vi "FG_FPGA_Interface.vi"(7 "Action":T1, 8 "error in":errorcluster) -> (0 "error out":errorcluster, 3 "FPGA VI Reference Out":refnum<k20>)   [LabVIEW 2014]
uses:
  Typedef_FPGA_Interface_Action.ctl
  <vilib>/FPGAPlugInAG/cRIO-9068/niLvFpga_Open_cRIO-9068.vi
  <vilib>/rvi/interface/common/dynamic/niFpgaDynamicAddResources.vi
  <vilib>/Utility/error.llb/Error Cluster From Error Code.vi
  <vilib>/rvi/errors/niLvFpgaAdjustHostInterfaceError.vi
  <vilib>/nisyscfg/Initialize (Control).vi
  <vilib>/nisyscfg/Find Hardware.vi
  <vilib>/FPGAPlugInAG/Dynamic/niLvFpga_Close_Dynamic.vi
  <vilib>/rvi/interface/nirviOpenFPGA/nirviOpenFPGA.xnode
  FPGA Bitfiles/Main FPGA 5-axis for Candy Packaging.lvbitx
  <vilib>/rvi/interface/nirviReadWriteControl/nirviReadWriteControl.xnode
  <vilib>/rvi/interface/nirviCloseFPGA/nirviCloseFPGA.xnode
  <vilib>/nisyscfg/nisyscfg.lvlib
  <vilib>/rvi/interface/Simulation/niFpgaSimulationCallBeginRW.vi
  NiFpgaLv.dll
panel:
  out "Numeric":i32
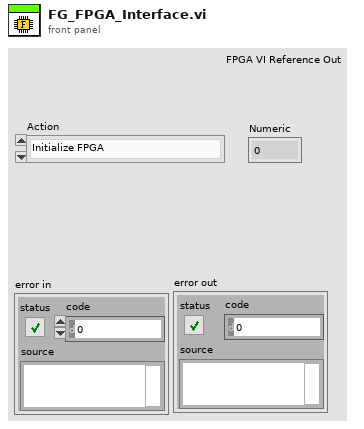
[diagram p1: front panel]
types:
  T1 = typedef "Typedef_FPGA_Interface_Action.ctl" = enum16{"Initialize FPGA", "Get FPGA Reference", "Close FPGA"}
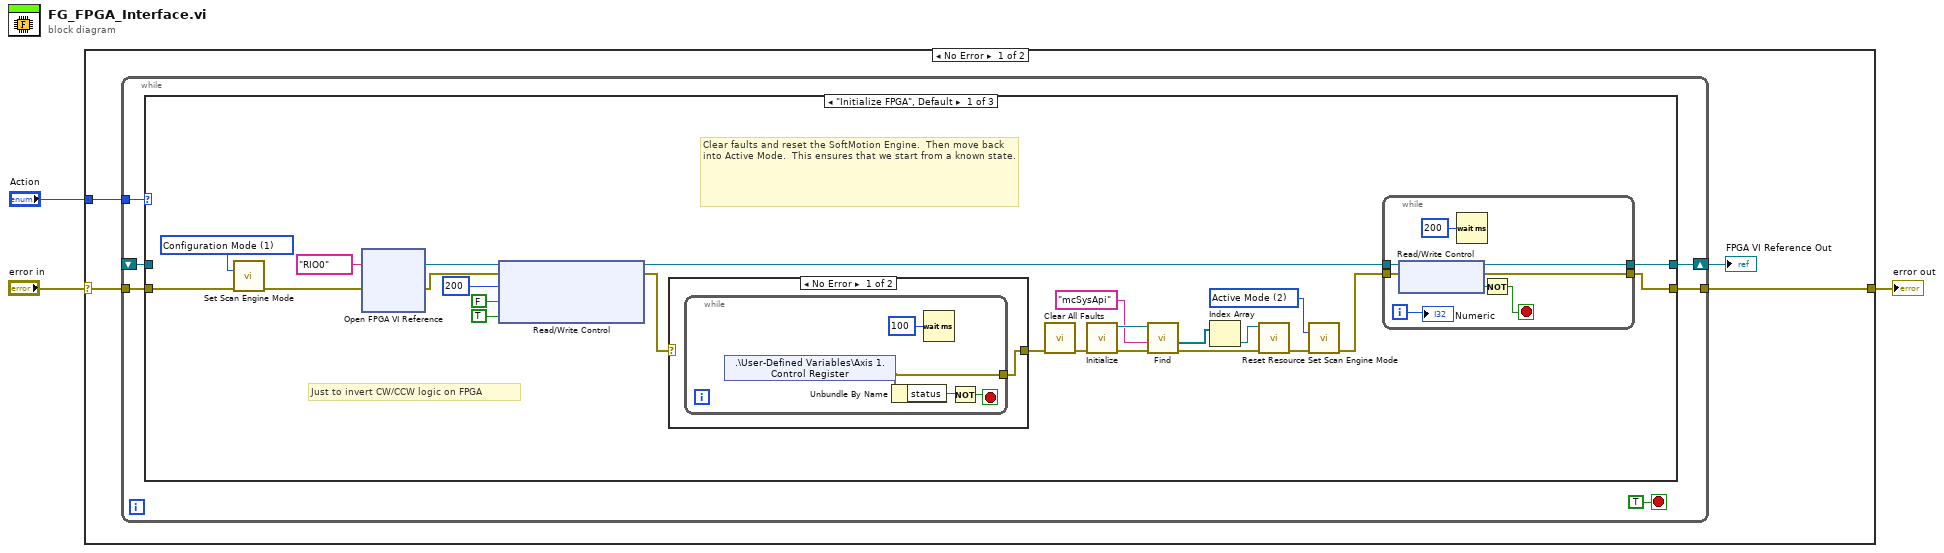
[diagram p0: block diagram]
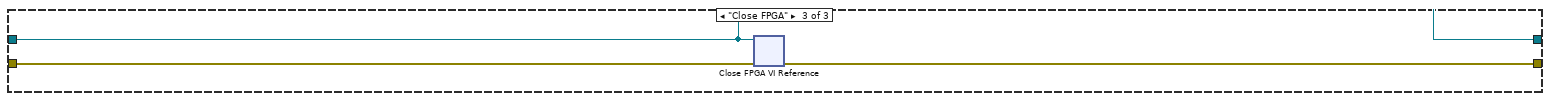
[diagram p4: hidden frame]
diagram:
  n1 = case shown="No Error" "error in" {
    selector: "error in" -> [w7 w57]
    tunnel: [w6 w57] -> w2
    tunnel: "Action" -> [w5 _]
    frame No Error {
      n2 = while {
        tunnel: w7 -> [w11]
        tunnel: w5 -> [w12]
        tunnel: [w10] -> w6
        shift-right: [w9] -> w4
        shift-left: _ -> [w8]
        stop <- TRUE stop-if-true
        n3 = case shown="\"Initialize FPGA\", Default" w12 {
          tunnel: w11 -> [w36 w52 w55]
          tunnel: [w17 w52 w56] -> w10
          tunnel: w8 -> [_ w53 w54]
          tunnel: [w18 w53 w54] -> w9
          frame "Initialize FPGA", Default {
            w20 = 2 items=["Configuration Mode"=1, "Active Mode"=2] ("mode (Active Mode)")
            w29 = 1 items=["Configuration Mode"=1, "Active Mode"=2] ("mode (Active Mode)")
            # "Just to invert CW/CCW logic on FPGA"
            # "Clear faults and reset the SoftMotion Engine.  Then move back into Active Mode.  This ensures that we start from a known state."
            n4 = call <vilib>:"Set Scan Engine Mode.vi"("mode (Active Mode)"=w29, "error in (no error)"=w36) -> ("error out"=w35:errorcluster)  [unwired: 13 in]
            n5 = xnode "Open FPGA VI Reference"("error in"=w35, "resource name"=tag "RIO0") -> ("FPGA VI Reference Out"=w15:refnum<k20>, "error out"=w16:errorcluster)
            n6 = xnode "Read/Write Control"("FPGA VI Reference In"=w15, "error in"=w16, "minimum pulse"=u16 200, "Invert direction?"=FALSE ("invert"), "STEP or CW? (T=STEP)"=TRUE) -> ("FPGA VI Reference Out"=w19:refnum<k20>, "error out"=w33:errorcluster)
            n7 = case shown="No Error" w33 {
              selector: w33 -> [_ w51]
              tunnel: [w46 w51] -> w34
              frame No Error {
                n8 = while {
                  tunnel: [w47] -> w46
                  stop <- w50 stop-if-true
                  n9 = shared-variable ".\\User-Defined Variables\\Axis 1.Control Register"() -> (error out=w47:errorcluster)  [unwired: 1 in, 1 out]
                  n10 = Unbundle By Name(w47) -> ("status"=w49:bool)
                  n11 = Wait (ms)(milliseconds to wait=u32 100) -> ()  [unwired: 1 out]
                  n12 = Not(x=w49) -> (.not. x?=w50:bool)
                }
              }
              frame Error {
              }
            }
            n13 = call <vilib>:"Clear All Faults.vi"("error in (no error)"=w34) -> ("error out"=w27:errorcluster)  [unwired: 10 in]
            n14 = call-poly <vilib>:"Initialize.vi"("error in (no error)"=w27) -> ("error out"=w21:errorcluster, "Session out"=w23:refnum<k21>)  [unwired: 8 in, 1 out]
            n15 = call-poly <vilib>:"Find.vi"("error in (no error)"=w21, "Experts"="mcSysApi" ("experts"), "Session in"=w23) -> ("error out"=w26:errorcluster, "Resources out"=w24:refnum<k20>[])  [unwired: 5 in, 2 out]
            n16 = Index Array(array=w24) -> (element=w25:refnum<k20>)  [unwired: 1 in]
            n17 = call <vilib>:"Reset Resource.vi"("error in (no error)"=w26, "Resource in"=w25) -> ("error out"=w28:errorcluster)  [unwired: 8 in, 1 out]
            n18 = call <vilib>:"Set Scan Engine Mode.vi"("mode (Active Mode)"=w20, "error in (no error)"=w28) -> ("error out"=w32:errorcluster)  [unwired: 13 in]
            n19 = while {
              tunnel: w32 -> [w45]
              tunnel: [w44] -> w17
              tunnel: w19 -> [w40]
              tunnel: [w39] -> w18
              i -> [w38]
              stop <- w41 stop-if-true
              n20 = xnode "Read/Write Control"("FPGA VI Reference In"=w40, "error in"=w45) -> ("FPGA VI Reference Out"=w39:refnum<k20>, "error out"=w44:errorcluster, "Sync is Fault"=w43:bool)
              n21 = Wait (ms)(milliseconds to wait=u32 200) -> ()  [unwired: 1 out]
              n22 = Not(x=w43) -> (.not. x?=w41:bool)
              "Numeric" <- w38
            }
          }
          frame "Get FPGA Reference" {
          }
          frame "Close FPGA" {
            n23 = xnode "Close FPGA VI Reference"("FPGA VI Reference In"=w54, "error in"=w55) -> ("error out"=w56:errorcluster)
          }
        }
      }
      "FPGA VI Reference Out" <- w4
    }
    frame Error {
    }
  }
  "error out" <- w2
